vi "Action.vi"(8 "error in (no error)":errorcluster, 10 "OOQMH in":refnum<class "OOQMH.lvclass">, 11 "Start Polling in":refnum<class "Start Polling.lvclass">) -> (0 "error out":errorcluster, 2 "OOQMH out":refnum<class "OOQMH.lvclass">, 3 "Start Polling out":refnum<class "Start Polling.lvclass">)   [LabVIEW 2024, in "OOQMH.lvlib" / "Start Polling.lvclass"]
uses:
  Start Polling.lvclass
  OOQMH/OOQMH.lvclass
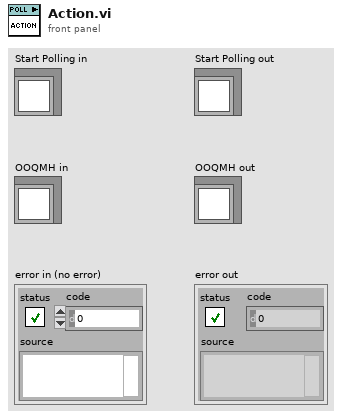
[diagram p1: front panel]
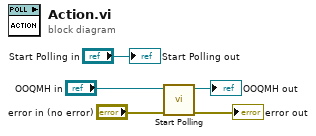
[diagram p0: block diagram]
diagram:
  n1 = call-dynamic "Start Polling.vi"("error in (no error)"="error in (no error)", "OOQMH in"="OOQMH in") -> ("error out"=→"error out":errorcluster, "OOQMH out"=→"OOQMH out":refnum<class "OOQMH.lvclass">)  [unwired: 8 in]
  "Start Polling out" <- "Start Polling in"
